vi "FGV_SQL_batch_ID_buffer.vi"(6 "connection reference":T2, 7 "options":T3, 8 "error_in":errorcluster, 9 "station":T1, 10 "BATCH_NUMBER":string, 11 "PART_NUMBER":string) -> (0 "error_out":errorcluster, 2 "PART_NUMBER exists?":bool, 3 "ID_out":string)   [LabVIEW 2020]
uses:
  FGV_SQL_batch_ID_buffer.ctl
  <vilib>/addons/database/Connection.llb/Conn ObjectReference.ctl
  STATION/station.ctl
  SQL_batch_ID_buffer_all_info.ctl
  <vilib>/addons/database/NI_Database_API.lvlib
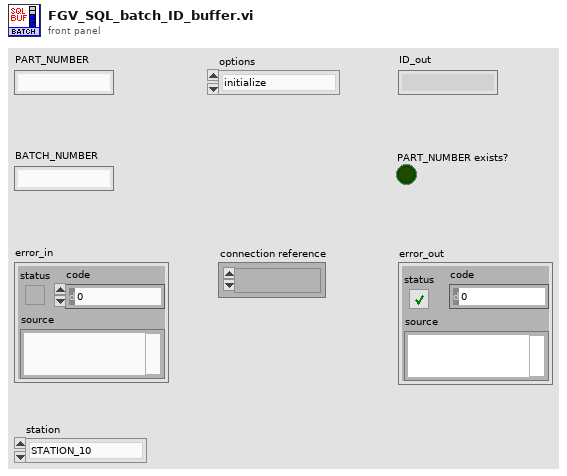
[diagram p1: front panel]
types:
  T1 = typedef "station.ctl" = enum16{"STATION_10", "STATION_20", "STATION_30", "STATION_40", "STATION_50", "STATION_60", "STATION_70", "STATION_80", "STATION_90", "STATION_100", "STATION_110", "STATION_120", "STATION_165", "MAIN"}
  T2 = typedef "NI_Database_API.lvlib/Conn ObjectReference.ctl" = refnum<k1>
  T3 = typedef "FGV_SQL_batch_ID_buffer.ctl" = enum16{"initialize", "get_ID_for_number"}
  T4 = typedef "SQL_batch_ID_buffer_all_info.ctl" = cluster{"BATCH_NUMBER_and_ID":string[][], "BATCH_NUMBER_and_ID_buffer_pos":i32, "BATCH_NUMBER_and_ID_buffer_max_size":i32}
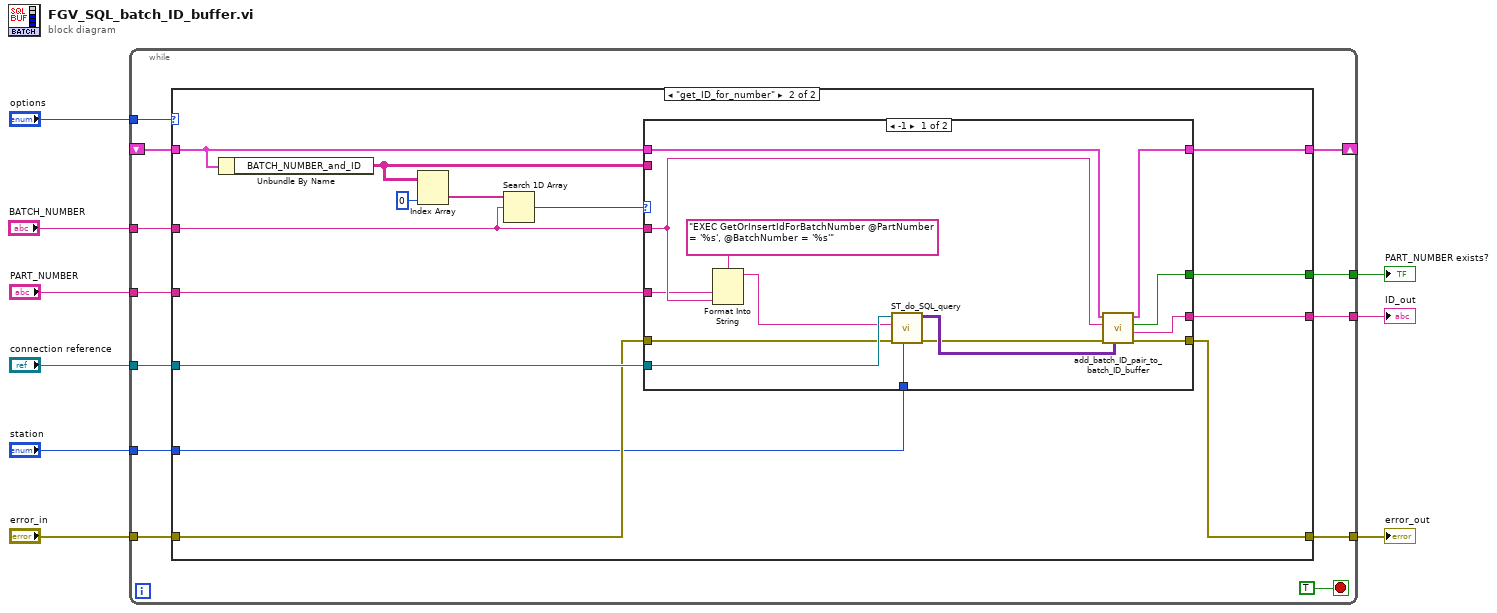
[diagram p0: block diagram]
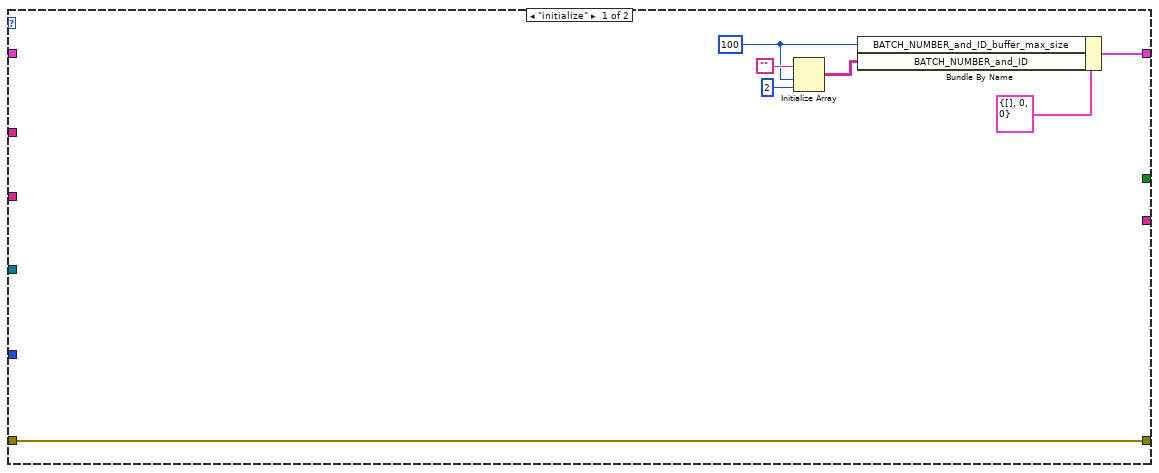
[diagram p2: hidden frame]
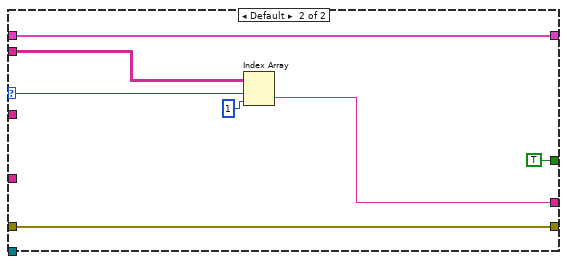
[diagram p3: hidden frame]
diagram:
  n1 = while {
    tunnel: "options" -> [w20]
    tunnel: [w19] -> w9
    tunnel: "error_in" -> [w18]
    shift-right: [w17] -> _
    shift-left: _ -> [w16]
    tunnel: "connection reference" -> [w14]
    tunnel: "PART_NUMBER" -> [w15]
    tunnel: [w13] -> w4
    tunnel: [w12] -> w3
    tunnel: "station" -> [w11]
    tunnel: "BATCH_NUMBER" -> [w10]
    stop <- TRUE stop-if-true
    n2 = case shown="\"get_ID_for_number\"" w20 {
      tunnel: [w28 w35] -> w19
      tunnel: w18 -> [w28 w36]
      tunnel: [w22 w33] -> w17
      tunnel: w16 -> [_ w34]
      tunnel: w15 -> [_ w29]
      tunnel: w14 -> [_ w37]
      tunnel: [_ w38] -> w13
      tunnel: [_ w32] -> w12
      tunnel: w11 -> [_ w31]
      tunnel: w10 -> [_ w30]
      frame "initialize" {
        w24 = 100 ("dimension size")
        n3 = Initialize Array("", w24, 2 ("dimension size")) -> (w27:string[][])
        n4 = Bundle By Name(cluster=T4 {"BATCH_NUMBER_and_ID"=[], "BATCH_NUMBER_and_ID_buffer_pos"=0, "BATCH_NUMBER_and_ID_buffer_max_size"=0} ("SQL_batch_ID_buffer_all_info"), "BATCH_NUMBER_and_ID_buffer_max_size"=w24, "BATCH_NUMBER_and_ID"=w27) -> (w22:T4)
      }
      frame "get_ID_for_number" {
        n5 = Unbundle By Name(w34) -> ("BATCH_NUMBER_and_ID"=w39:string[][])
        n6 = Index Array(array=w39, index (col)=0 ("disabled index (col)")) -> (element=w41:string[])  [unwired: 1 in]
        n7 = Search 1D Array(1D array=w41, element=w30) -> (index of element=w40:i32)  [unwired: 1 in]
        n8 = case shown="-1" w40 {
          selector: w40 -> [_ w63]
          tunnel: w39 -> [_ w62]
          tunnel: [w52 w60] -> w38
          tunnel: w37 -> [w51 _]
          tunnel: w30 -> [w44 _]
          tunnel: w36 -> [w48 w59]
          tunnel: [w55 w59] -> w35
          tunnel: w34 -> [w54 w58]
          tunnel: [w53 w58] -> w33
          tunnel: [w50 TRUE ("Part exists?")] -> w32
          tunnel: w31 -> [w46 _]
          tunnel: w29 -> [w43 _]
          frame -1 {
            n9 = Format Into String(format string="EXEC GetOrInsertIdForBatchNumber @PartNumber = '%s', @BatchNumber = '%s'", w43, w44) -> (resulting string=w47:string)  [unwired: 2 in, 1 out]
            n10 = call "ST_do_SQL_query.vi"("station"=w46, "error_in"=w48, "SQL_query"=w47, "SQL_connection_reference"=w51) -> ("error_out"=w45:errorcluster, "recordset_out"=w49:variant[][])  [unwired: 6 in]
            n11 = call "add_batch_ID_pair_to_batch_ID_buffer.vi"("recordset_in"=w49, "error_in"=w45, "BATCH_NUMBER"=w44, "SQL_batch_ID_buffer_all_info_in"=w54) -> ("error_out"=w55:errorcluster, "BATCH_ID_out"=w52:string, "PART_NUMBER exists?"=w50:bool, "SQL_batch_ID_buffer_all_info_out"=w53:T4)  [unwired: 4 in]
          }
          frame Default {
            n12 = Index Array(array=w62, index (row)=w63, index (col)=1 ("disabled index (col)")) -> (element=w60:string)
          }
        }
      }
    }
  }
  "error_out" <- w9
  "ID_out" <- w4
  "PART_NUMBER exists?" <- w3
